vi "Release Local References.vi"(8 "error in (no error)":errorcluster, 11 "Selection in":refnum<class "Selection.lvclass">) -> (0 "error out":errorcluster)   [LabVIEW 2015, in "LV Image Editor Framework.lvlib" / "Selection.lvclass"]
uses:
  Selection.lvclass
  Selection.lvclass/Selection.ctl
  Shape/Shape.lvclass
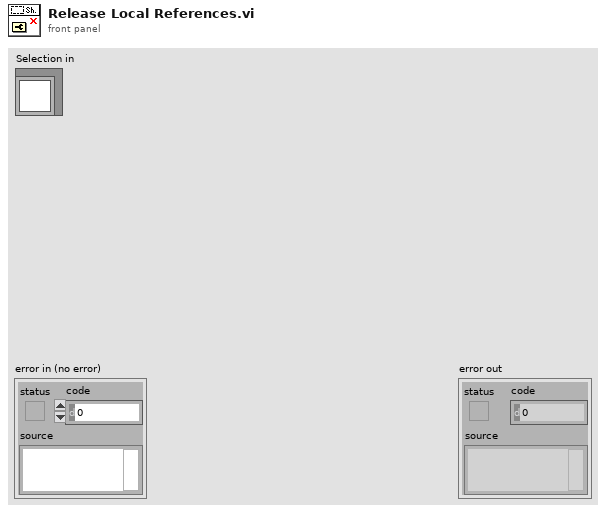
[diagram p1: front panel]
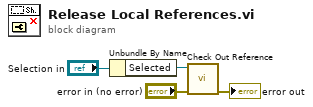
[diagram p0: block diagram]
diagram:
  n1 = Unbundle By Name("Selection in") -> ("Selected"=w3:refnum<data-value>)
  n2 = call "Check Out Reference.vi"("error in (no error)"="error in (no error)", "Shape Reference"=w3) -> ("error out"=→"error out":errorcluster)  [unwired: 9 in]
